vi "俄罗斯方块-绘制文本.vi"(0 "输入图片":picture, 5 "最高分数":u32, 7 "最多行数":u32, 9 "分数":u32, 11 "行数":u32, 12 "结束状态":bool, 13 "开始/暂停":bool) -> (4 "输出图片":picture)   [LabVIEW 2021]
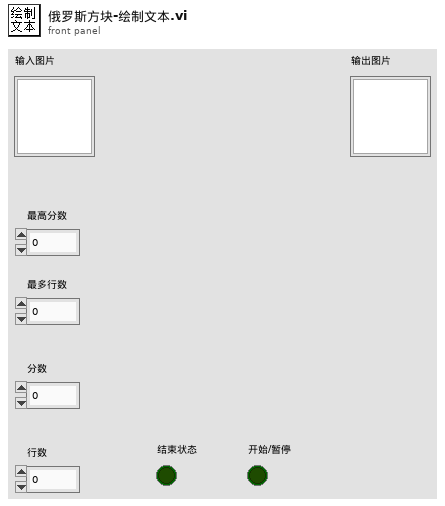
[diagram p1: front panel]
types:
  T1 = cluster{"Font Name:":string, "Size":i16, "Strikeout?":bool, "Italic?":bool, "Underline?":bool, "Outline?":bool, "Shadow?":bool, "Bold?":bool}
  T2 = cluster{"horizontal":enum16{"left", "center", "right"}, "vertical":enum16{"top", "center", "bottom"}}
  T3 = cluster{"Width":i16, "Style":enum32{"Solid", "Dash", "Dot", "DashDot", "DashDotDot"}}
  T4 = enum16{"User-specified Font", "Application Font", "System Font", "Dialog Font"}
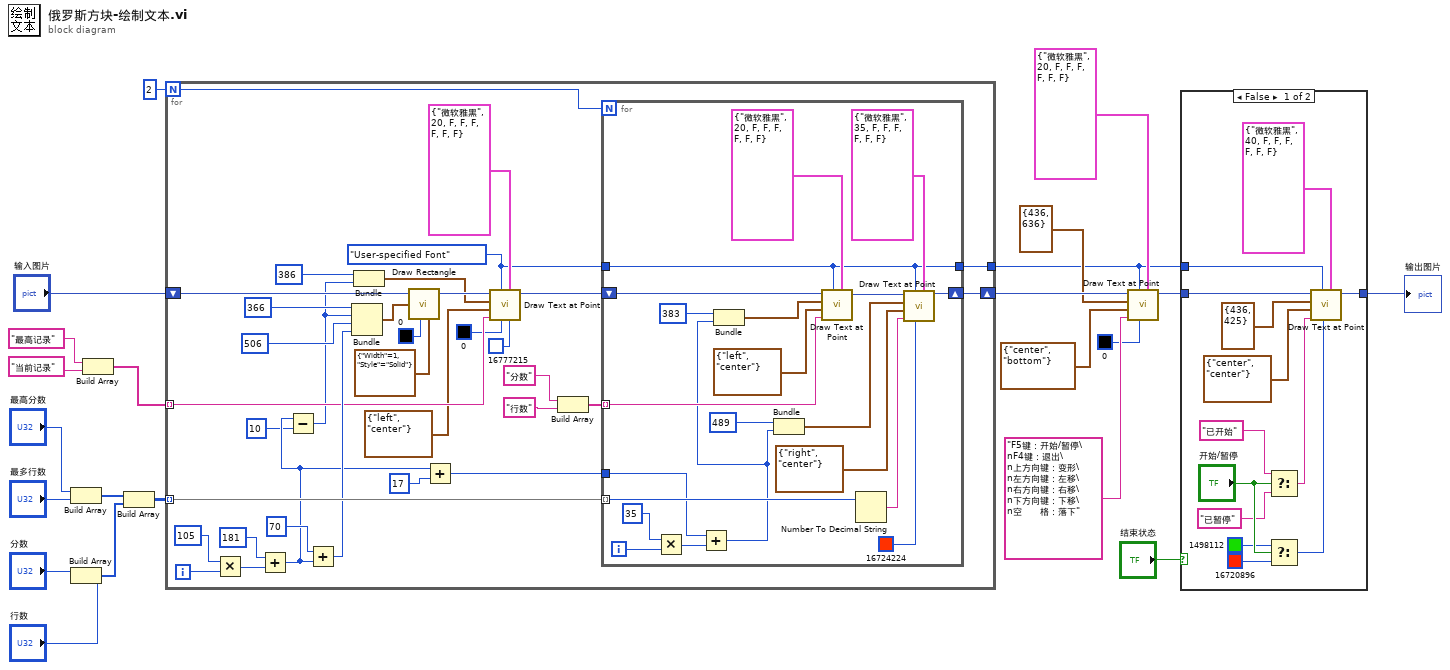
[diagram p0: block diagram]
diagram:
  n1 = Build Array("最高分数", "最多行数") -> (w12:u32[])
  n2 = Build Array("分数", "行数") -> (w13:u32[])
  n3 = Build Array("最高记录", "当前记录") -> (w20:string[])
  n4 = Build Array(w12, w13) -> (w19:u32[][])
  n5 = for {
    N: 2 -> [w54]
    tunnel: w20 -> [w30] mode=indexing
    tunnel: w19 -> [w56] mode=indexing
    shift-right: [w55] -> w7
    shift-left: "输入图片" -> [w53]
    tunnel: [w23] -> w2
    i -> [w40]
    w46 = T4."User-specified Font" ("desired font(Application)")
    n6 = Multiply(x=105, y=w40) -> (x*y=w43:i32)
    n7 = Add(x=181 ("y"), y=w43) -> (x+y=w35:i32)
    n8 = Subtract(x=w35, y=10) -> (x-y=w25:i32)
    n9 = Add(x=70, y=w35) -> (x+y=w39:i32)
    n10 = Bundle("Width"=i16 366, w25, "Width"=i16 506, w39) -> (w52:cluster{"Width":i16, i32, "Width":i16, i32})  [unwired: 1 in]
    n11 = Bundle("Width"=i16 386, w25) -> (w26:cluster{"Width":i16, i32})  [unwired: 1 in]
    n12 = call <vilib>:"Draw Rectangle.vi"("picture"=w53, "rect"=w52, "color(black)"=u32 0, "pen"=T3 {"Width"=1, "Style"=enum."Solid"}) -> ("new picture"=w49:picture)  [unwired: 5 in]
    n13 = Add(x=w35, y=17) -> (x+y=w36:i32)
    n14 = call <vilib>:"Draw Text at Point.vi"("BG color(transparent)"=u32 16777215, "[user-specified font]"=T1 {"Font Name:"="微软雅黑", "Size"=20, "Strikeout?"=FALSE, "Italic?"=FALSE, "Underline?"=FALSE, "Outline?"=FALSE, "Shadow?"=FALSE, "Bold?"=FALSE}, "text color(black)"=u32 0, "desired font(Application)"=w46, "text"=w30, "alignment(left, top)"=T2 {"horizontal"=enum."left", "vertical"=enum."center"}, "origin"=w26, "picture"=w49) -> ("new picture"=w48:picture)  [unwired: 2 in, 1 out]
    n15 = Build Array("分数", "行数") -> (w31:string[])
    n16 = for {
      N: w54 -> [_]
      tunnel: w31 -> [w69] mode=indexing
      tunnel: w56 -> [w72] mode=indexing
      shift-right: [w60] -> w55
      shift-left: w48 -> [w77]
      tunnel: w46 -> [w57]
      tunnel: w36 -> [w58]
      tunnel: [w57] -> w23
      i -> [w65]
      n17 = Multiply(x=35, y=w65) -> (x*y=w63:i32)
      n18 = Add(x=w58, y=w63) -> (x+y=w61:i32)
      n19 = Bundle(383, w61) -> (w68:cluster{i32, i32})  [unwired: 1 in]
      n20 = Bundle(489, w61) -> (w66:cluster{i32, i32})  [unwired: 1 in]
      n21 = call <vilib>:"Draw Text at Point.vi"("[user-specified font]"=T1 {"Font Name:"="微软雅黑", "Size"=20, "Strikeout?"=FALSE, "Italic?"=FALSE, "Underline?"=FALSE, "Outline?"=FALSE, "Shadow?"=FALSE, "Bold?"=FALSE}, "desired font(Application)"=w57, "text"=w69, "alignment(left, top)"=T2 {"horizontal"=enum."left", "vertical"=enum."center"}, "origin"=w68, "picture"=w77) -> ("new picture"=w74:picture)  [unwired: 4 in, 1 out]
      n22 = Number To Decimal String(number=w72) -> (decimal integer string=w73:string)  [unwired: 1 in]
      n23 = call <vilib>:"Draw Text at Point.vi"("[user-specified font]"=T1 {"Font Name:"="微软雅黑", "Size"=35, "Strikeout?"=FALSE, "Italic?"=FALSE, "Underline?"=FALSE, "Outline?"=FALSE, "Shadow?"=FALSE, "Bold?"=FALSE}, "text color(black)"=u32 16724224, "desired font(Application)"=w57, "text"=w73, "alignment(left, top)"=T2 {"horizontal"=enum."right", "vertical"=enum."center"}, "origin"=w66, "picture"=w74) -> ("new picture"=w60:picture)  [unwired: 3 in, 1 out]
    }
  }
  n24 = call <vilib>:"Draw Text at Point.vi"("[user-specified font]"=T1 {"Font Name:"="微软雅黑", "Size"=20, "Strikeout?"=FALSE, "Italic?"=FALSE, "Underline?"=FALSE, "Outline?"=FALSE, "Shadow?"=FALSE, "Bold?"=FALSE}, "text color(black)"=u32 0, "desired font(Application)"=w2, "text"="F5键：开始/暂停\nF4键：退出\n上方向键：变形\n左方向键：左移\n右方向键：右移\n下方向键：下移\n空　　格：落下", "alignment(left, top)"=T2 {"horizontal"=enum."center", "vertical"=enum."bottom"}, "origin"=cluster{"x":i16, "y":i16} {"x"=436, "y"=636}, "picture"=w7) -> ("new picture"=w4:picture)  [unwired: 3 in, 1 out]
  n25 = case shown="False" "结束状态" {
    tunnel: w4 -> [w90 w91]
    tunnel: [w89 w91] -> w3
    tunnel: w2 -> [w88 _]
    frame False {
      n26 = Select(t="已开始" ("text"), s="开始/暂停", f="已暂停" ("text")) -> (s? t:f=w79:string)
      n27 = Select(t=u32 1498112 ("text color(black)"), s="开始/暂停", f=u32 16720896 ("text color(black)")) -> (s? t:f=w78:u32)
      n28 = call <vilib>:"Draw Text at Point.vi"("[user-specified font]"=T1 {"Font Name:"="微软雅黑", "Size"=40, "Strikeout?"=FALSE, "Italic?"=FALSE, "Underline?"=FALSE, "Outline?"=FALSE, "Shadow?"=FALSE, "Bold?"=FALSE}, "text color(black)"=w78, "desired font(Application)"=w88, "text"=w79, "alignment(left, top)"=T2 {"horizontal"=enum."center", "vertical"=enum."center"}, "origin"=cluster{"x":i16, "y":i16} {"x"=436, "y"=425}, "picture"=w90) -> ("new picture"=w89:picture)  [unwired: 3 in, 1 out]
    }
    frame True {
    }
  }
  "输出图片" <- w3
